vi "Pre Launch Init.vi"(11 "DAQ AI in":refnum<class "DAQ AI.lvclass">) -> (0 "error out":errorcluster, 3 "DAQ AI out":refnum<class "DAQ AI.lvclass">)   [LabVIEW 2020, in "DAQ AI.lvlib" / "DAQ AI.lvclass"]
doc: "<p>(<strong>Filename</strong>: <span class=\"dnl\">Actor Framework.lvlib:Actor.lvclass:Pre Launch Init.vi</span>)</p>\n<p>Defines behavior that occurs after the <a href=\"nihelplauncher://docs/csh?context=lvcore_lvcomm_af_launch_nested_actor\">Launch Nested Actor</a> method is invoked but before the actor's Actor Core method begins running.</p>\n<p>By default, this method does nothing. A descendant class may override it to define behavior.</p>"
uses:
  DAQ AI.lvclass
  DAQ AI.lvclass/DAQ AI.ctl
  <vilib>/ActorFramework/Actor/Actor.lvclass
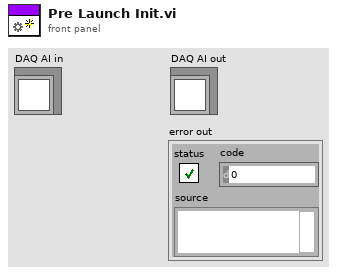
[diagram p1: front panel]
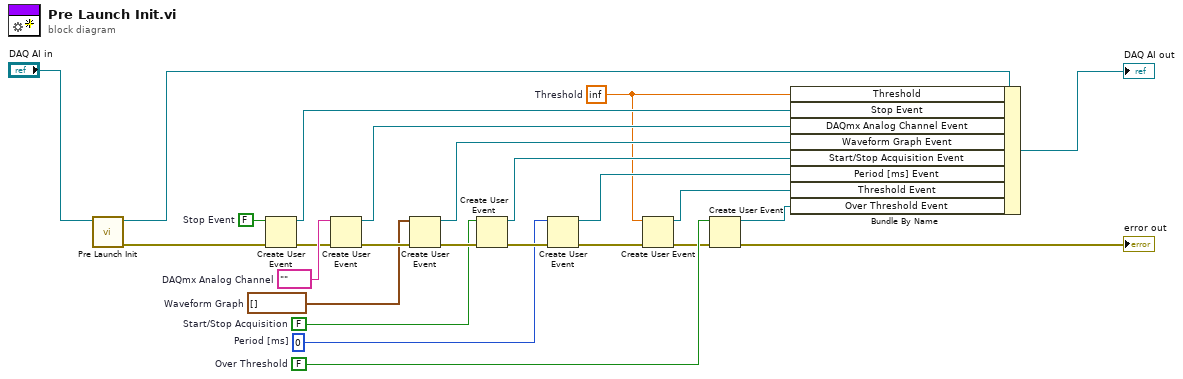
[diagram p0: block diagram]
diagram:
  w4 = FALSE  # Over Threshold
  w7 = inf  # Threshold
  w12 = FALSE  # Stop Event
  w19 = tag ""  # DAQmx Analog Channel
  w17 = waveform(dbl)[] []  # Waveform Graph
  w15 = FALSE  # Start/Stop Acquisition
  w14 = 0  # Period [ms]
  n1 = call-parent "Pre Launch Init.vi"("Actor in"="DAQ AI in") -> ("error out"=w11:errorcluster, "Actor out"=w24:refnum<class "DAQ AI.lvclass">)  [unwired: 9 in]
  n2 = Create User Event(user event datatype=w12, error in=w11) -> (user event=w9:refnum<user-event>, error out=w10:errorcluster)
  n3 = Create User Event(user event datatype=w19, error in=w10) -> (user event=w18:refnum<user-event>, error out=w22:errorcluster)
  n4 = Create User Event(user event datatype=w17, error in=w22) -> (user event=w16:refnum<user-event>, error out=w21:errorcluster)
  n5 = Create User Event(user event datatype=w15, error in=w21) -> (user event=w8:refnum<user-event>, error out=w20:errorcluster)
  n6 = Create User Event(user event datatype=w14, error in=w20) -> (user event=w13:refnum<user-event>, error out=w6:errorcluster)
  n7 = Create User Event(user event datatype=w7, error in=w6) -> (user event=w5:refnum<user-event>, error out=w3:errorcluster)
  n8 = Create User Event(user event datatype=w4, error in=w3) -> (user event=w1:refnum<user-event>, error out=→"error out":errorcluster)
  n9 = Bundle By Name(cluster=w24, "Threshold"=w7, "Stop Event"=w9, "DAQmx Analog Channel Event"=w18, "Waveform Graph Event"=w16, "Start/Stop Acquisition Event"=w8, "Period [ms] Event"=w13, "Threshold Event"=w5, "Over Threshold Event"=w1) -> (→"DAQ AI out":refnum<class "DAQ AI.lvclass">)
